vi "GlobalClicksHeight_FBL.vi"() -> ()   [LabVIEW 2017]
panel:
  out "Setpoint (A)":dbl=100.0
  out "Current (pA)":dbl
  in  "Found Surface?":bool
  out "Surface Location (nm)":dbl
  in  "Starting Height?":bool
  in  "Clicks and Height":bool
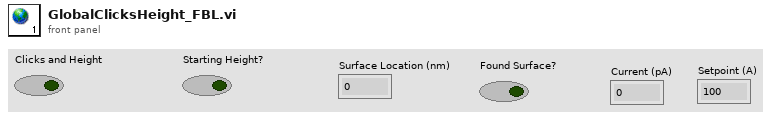
[diagram p1: front panel]
diagram:
